vi "Save Data (All).vi"(0 "Filepath":path, 1 "DataRowsSaved":i32, 2 "DataRowIndex":i32, 3 "Data":string[][](array[string]), 11 "Error In":errorcluster) -> (15 "Error Out":errorcluster)   [LabVIEW 2013]
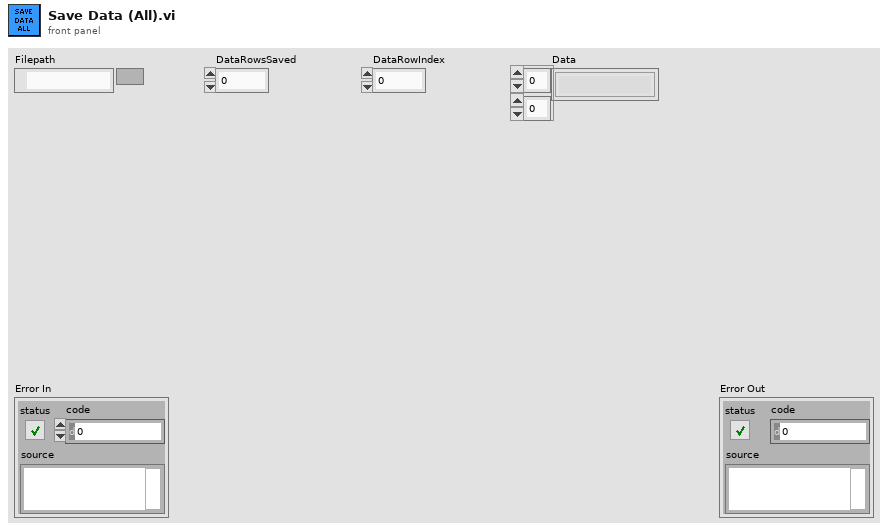
[diagram p1: front panel]
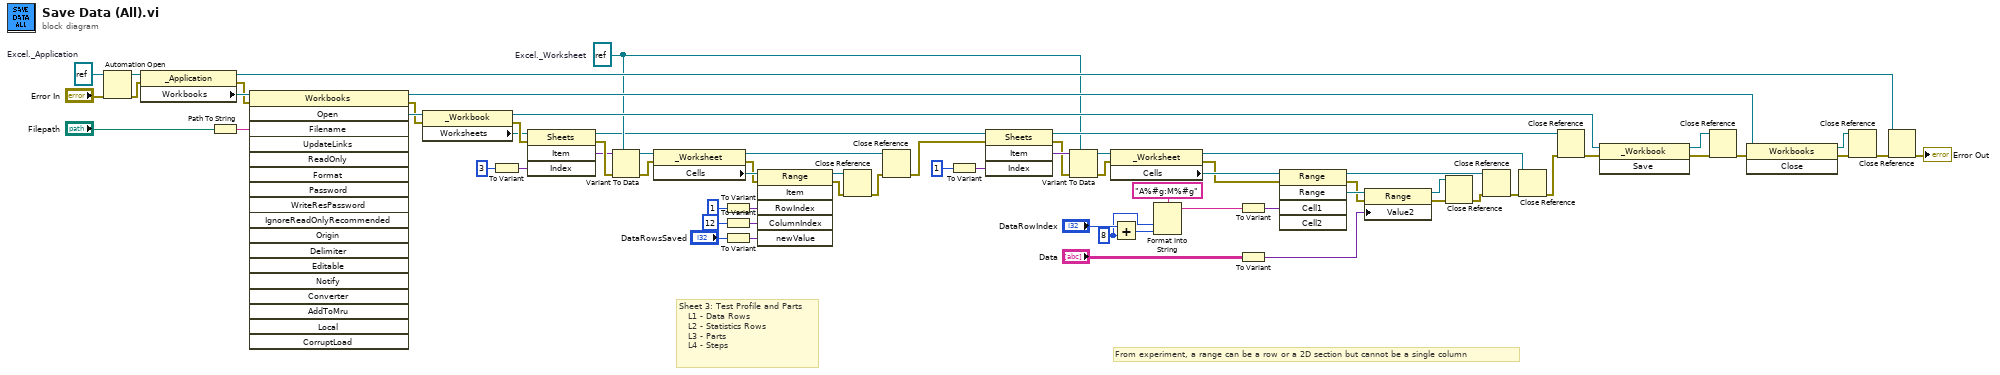
[diagram p0: block diagram]
diagram:
  w1 = 8 ("y")
  w42 = refnum<k7> refnum  # Excel._Worksheet
  w67 = refnum<k7> refnum  # Excel._Application
  # "Sheet 3: Test Profile and Parts\n   L1 - Data Rows\n   L2 - Statistics Rows\n   L3 - Parts\n   L4 - Steps"
  # "From experiment, a range can be a row or a 2D section but cannot be a single column"
  n1 = Automation Open(error in (no error)="Error In", Automation Refnum=w67) -> (Automation Refnum=w68:refnum<k7>, error out=w69:errorcluster)  [unwired: 2 in]
  n2 = property class="_Application"(reference=w68, error in=w69) -> (reference out=w60:refnum<k7>, error out=w61:errorcluster, "Workbooks"=w70:refnum<k7>)
  n3 = Path To String(path="Filepath") -> (string=w57:string)
  n4 = invoke class="Workbooks" method="Open"(reference=w70, error in=w61, "Filename"=w57) -> (reference out=w64:refnum<k7>, error out=w59:errorcluster, "Open"=w66:refnum<k7>)  [unwired: 15 in, 15 out]
  n5 = property class="_Workbook"(reference=w66, error in=w59) -> (reference out=w53:refnum<k7>, error out=w45:errorcluster, "Worksheets"=w44:refnum<k7>)
  n6 = To Variant(anything=3) -> (Variant=w46:variant)
  n7 = invoke class="Sheets" method="Item"(reference=w44, error in=w45, "Index"=w46) -> (reference out=w38:refnum<k7>, error out=w48:errorcluster, "Item"=w47:variant)  [unwired: 1 in, 1 out]
  n8 = Variant To Data(error in=w48, type=w42, Variant=w47) -> (data=w49:refnum<k7>, error out=w50:errorcluster)
  n9 = property class="_Worksheet"(reference=w49, error in=w50) -> (reference out=w37:refnum<k7>, error out=w4:errorcluster, "Cells"=w5:refnum<k7>)
  n10 = To Variant(anything=1) -> (Variant=w33:variant)
  n11 = To Variant(anything=12) -> (Variant=w34:variant)
  n12 = To Variant(anything="DataRowsSaved") -> (Variant=w41:variant)
  n13 = invoke class="Range" method="Item"(reference=w5, error in=w4, "RowIndex"=w33, "ColumnIndex"=w34, "newValue"=w41) -> (reference out=w3:refnum<k7>, error out=w2:errorcluster)  [unwired: 1 in, 4 out]
  n14 = Close Reference(reference=w3, error in (no error)=w2) -> (error out=w36:errorcluster)
  n15 = Close Reference(reference=w37, error in (no error)=w36) -> (error out=w35:errorcluster)
  n16 = To Variant(anything=1) -> (Variant=w27:variant)
  n17 = invoke class="Sheets" method="Item"(reference=w38, error in=w35, "Index"=w27) -> (reference out=w51:refnum<k7>, error out=w25:errorcluster, "Item"=w26:variant)  [unwired: 1 in, 1 out]
  n18 = Variant To Data(error in=w25, type=w42, Variant=w26) -> (data=w24:refnum<k7>, error out=w23:errorcluster)
  n19 = property class="_Worksheet"(reference=w24, error in=w23) -> (reference out=w21:refnum<k7>, error out=w17:errorcluster, "Cells"=w18:refnum<k7>)
  n20 = Add(x="DataRowIndex", y=w1) -> (x+y=w14:i32)
  n21 = Format Into String(format string="A%#g:M%#g", w1, w14) -> (resulting string=w7:string)  [unwired: 2 in, 1 out]
  n22 = To Variant(anything=w7) -> (Variant=w12:variant)
  n23 = To Variant(anything="Data") -> (Variant=w10:variant)
  n24 = invoke class="Range" method="Range"(reference=w18, error in=w17, "Cell1"=w12) -> (reference out=w20:refnum<k7>, error out=w11:errorcluster, "Range"=w13:refnum<k7>)  [unwired: 2 in, 2 out]
  n25 = property class="Range"(reference=w13, error in=w11, "Value2"=w10) -> (reference out=w9:refnum<k7>, error out=w8:errorcluster)
  n26 = Close Reference(reference=w9, error in (no error)=w8) -> (error out=w19:errorcluster)
  n27 = Close Reference(reference=w20, error in (no error)=w19) -> (error out=w22:errorcluster)
  n28 = Close Reference(reference=w21, error in (no error)=w22) -> (error out=w52:errorcluster)
  n29 = Close Reference(reference=w51, error in (no error)=w52) -> (error out=w58:errorcluster)
  n30 = invoke class="_Workbook" method="Save"(reference=w53, error in=w58) -> (reference out=w54:refnum<k7>, error out=w55:errorcluster)  [unwired: 1 in, 1 out]
  n31 = Close Reference(reference=w54, error in (no error)=w55) -> (error out=w56:errorcluster)
  n32 = invoke class="Workbooks" method="Close"(reference=w64, error in=w56) -> (reference out=w63:refnum<k7>, error out=w62:errorcluster)  [unwired: 1 in, 1 out]
  n33 = Close Reference(reference=w63, error in (no error)=w62) -> (error out=w65:errorcluster)
  n34 = Close Reference(reference=w60, error in (no error)=w65) -> (error out=→"Error Out":errorcluster)
